vi "Choreo_Util_AllianceFlipGetFlipper.vi"() -> (3 "Flipper":T1)   [LabVIEW 2019, in "ChoreoLib.lvlib"]
doc: "trajectory, mirrored across the field midline.\n\nInputs: \n - ChoreoTrajectory - cluster - Input trajectory\n\nOutputs:\n - Flipped Trajectory - cluster - trajectory, mirrored across the field midline."
uses:
  ChoreoLib.lvlib
  ENum/Choreo_Util_AllianceFlipType.ctl
  Choreo_Choreo_Globals.vi
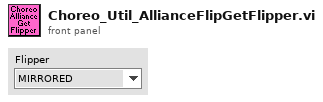
[diagram p1: front panel]
types:
  T1 = typedef "ChoreoLib.lvlib/Choreo_Util_AllianceFlipType.ctl" = enum16{"MIRRORED", "ROTATE_AROUND"}
  T2 = cluster{"Year":i32, "AllianceFlipType":T1, "FieldLength":dbl, "FieldWidth":dbl}
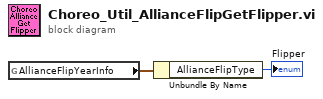
[diagram p0: block diagram]
diagram:
  n1 = global read "Choreo_Choreo_Globals.vi" "AllianceFlipYearInfo"() -> (w2:T2)
  n2 = Unbundle By Name(w2) -> ("AllianceFlipType"=→"Flipper":T1)
